vi "GetLeCroy_SaveToFile_25.vi"(1 "Digitizer Settings":T8={"Digitizer delay (us) "=0.0, "rf points per line"=2048, "lines per plane"=128, "Samp Rate (Hz)"=100000000.0, "Additional dig delay (us)"=0.0, "Voltage Scale"=0.4, "Pre-Looks"=0, "Offset delay (us)"=0.0, "bits A/D"=8, "Avg Num"=1, "DigTimeOut"=5.0, "Rel Dig Delay"=0.0, "Dig Ch"=0, "LeCroyCluster"={"LeCroy Channels"=[TRUE, FALSE, FALSE, FALSE], "LC read pt offset"=0.0, "Sweep Avg"=FALSE}, "Main Digitizer"=enum."NI Digitizer", "Dig Config"=enum."Single channel", "Digitizer ID Cluster"={"Acqiris/Alazar/SP ID"=[], "NI Instr Handles"=[], "LeCroy VISA"="", "GaGe Handle"={"Handle"=0, "Sample size"=0, "Resolution"=0, "Offset"=0, "Channels"=0, "Boards"=0}, "ATS Ref"="ATS9350", "Acqiris Address"=["PCI::INSTR0"], "ADQRef"=refnum, "adq_cu_ptr"=refnum}, "Trigger Settings"={"Trig Source"=1, "Trig Coupling"=0, "Trig Slope"=0, "Level (mV)"=1500.0}, "Bulk Acq"=FALSE, "Bulk Start Indexes"=[], "Data Ref RF"=refnum, "NI ID/Channel"=[], "Total Dig CH"=1, "Xtra Ann Trig delay (us)"=10.0, "Fix Z Delay?"=FALSE, "One Way Transmission?"=FALSE, "Data Ref Log"=refnum} {"Trigger Settings"."Trig Slope" items=["Positive", "Negative"]; "Trigger Settings"."Level (mV)" format="%.2f"; "Trigger Settings"."Trig Coupling" items=["DC 1 MOhm", "AC 1 MOhm", "DC 50 Ohm", "AC 50 Ohm"]; "Trigger Settings"."Trig Source" items=["Chan 1", "External"]; "Rel Dig Delay" format="%.2f"; "DigTimeOut" format="%.2f"; "Avg Num" min=1; "Offset delay (us)" format="%.2f"; "Additional dig delay (us)" format="%.2f"; "Digitizer delay (us)" format="%.2f"}, 4 "Ann Array Params":T1={"Synth Foc?"=FALSE, "Focal Zones"=41, "Switch T/R"=0, "Trans Geometry (mm)"={"Transducer"=0, "Geo Focus"=12.0, "a (radius)"=3.0, "# of rings"=5, "kerf space "=0.1, "Center Freq"=12.0}, "Sub Ap Excite?"=FALSE, "Full Array Scan?"=FALSE, "Xmt/Rcv"={"XMIT"=[TRUE, TRUE, TRUE, TRUE, TRUE], "RCV"=[TRUE, TRUE, TRUE, TRUE, TRUE]}, "PulseSpacing (us)"=0.0, "Xmit Ring"=0, "XMIT CHS"=0, "RCV CHS"=0, "GPU?"=FALSE, "Save TIFF?"=FALSE, "downfactor"=1, "RCV 1CH"=0} {"RCV 1CH" items=["All", "1", "2", "3", "4", "5"]; "Trans Geometry (mm)"."Transducer" items=["6D 12R 40 MHz"=0, "10D 31R 20 MHz"=1, "10D 23R 20 MHz"=2, "6D 23R 40 MHz"=3, "4.5D 10.7R 40 MHz"=4, "9D 23.5R 20 MHz"=5, "9D 25.8R 20MHz"=6, "Enter"=99]; "Switch T/R" min=1 max=5 step=1}, 5 "errorin":errorcluster, 6 "File Array":string[](array[string]), 7 "Motion Settings":T4={"No Motion?"=FALSE, "Motion System"=enum."NI 735x", "Motion Bd ID"=1, "Motion Profile"="SMAC1", "# Axis"=1, "Reverse Z axis?"=TRUE, "SMAC Axis"=0, "scan pair"=enum."y-(x) scan", "RT fps"=6.0, "Steps per mm"=[1000, 1000, 1000, 1000], "Motor Parameters"={"velocity ct/s"=[10000.0, 10000.0, 10000.0, 50000.0], "accel ct/s^2"=[50000.0, 50000.0, 50000.0, 200000.0]}, "One Way Scan"=FALSE, "Reverse One Way Scan"=FALSE, "Global Position (mm)"=[], "Plane"=0, "Distance between\nscan lines (um)"=0.0, "Distance between\nscan planes (um)"=0.0, "number of scan planes"=1, "Total steps in line"=0, "Xtra plane\ndistance  (um)"=100, "Xtra planes "=1, "Add Axis"=FALSE, "overshoot cts"=200, "BKPT Shift"=0, "Scan Start Time (ms)"=0, "ESP VISA"="GPIB::1::INSTR", "3rd Axis"=1, "GL Ref Out"=refnum, "Galil Address"=""} {"3rd Axis" items=["x", "y", "z", "w"]; "Xtra planes" min=1; "Xtra plane\ndistance  (um)" min=0; "Distance between\nscan planes (um)" format="%.2f"; "Distance between\nscan lines (um)" format="%.2f"; "SMAC Axis" items=["None"=0, "Axis 1"=1, "Axis 2"=2, "Axis 3"=3, "Axis 4"=4, "Axis 5"=5, "Axis 6"=6, "Axis 7"=7, "Axis 8"=8, "Vector Space 1"=17, "Vector Space 2"=18, "Vector Space 3"=19, "Vector Space 4"=20]; "Motion Bd ID" min=1 max=32 step=1}, 8 "lines per plane":i32, 11 "Reverse?":bool) -> (12 "Gain Array":T12(array[cluster]), 13 "Raw VGain (scale)":dbl, 15 "VGain (dB)":dbl, 19 "error out":errorcluster)   [LabVIEW 2022 SP3]
uses:
  -DigitizerRoutines/DigitizerSettings.ctl
  -DigitizerRoutines/Digitizer.ctl
  -DigitizerRoutines/DigConfig.ctl
  -DigitizerRoutines/DigitizerID.ctl
  C:/Windows/System32/ADQAPI_dotNet_helper.dll
  Motion Controllers/NI_controller/-NI_MotionRoutines/MotionParameters.ctl
  Motion Controllers/NI_controller/-NI_MotionRoutines/MotionSys.ctl
  Motion Controllers/-MotionRoutines/ScanAxis.ctl
  Motion Controllers/-MotionRoutines/3rdAxis.ctl
  Annular Array/-AnnularRoutines/AnnularArray.ctl
  Annular Array/-AnnularRoutines/TransGeometry.ctl
  Annular Array/-AnnularRoutines/ArrayGeometry.ctl
  Motion Controllers/-MotionRoutines/MotionGlobals.vi
  -ScanSystem/DataHandling/ReverseData.vi
panel:
  out "read time":u32
  out "save time":u32
  out "Numeric":i32
  # "1-D and 2-D B scan settings"
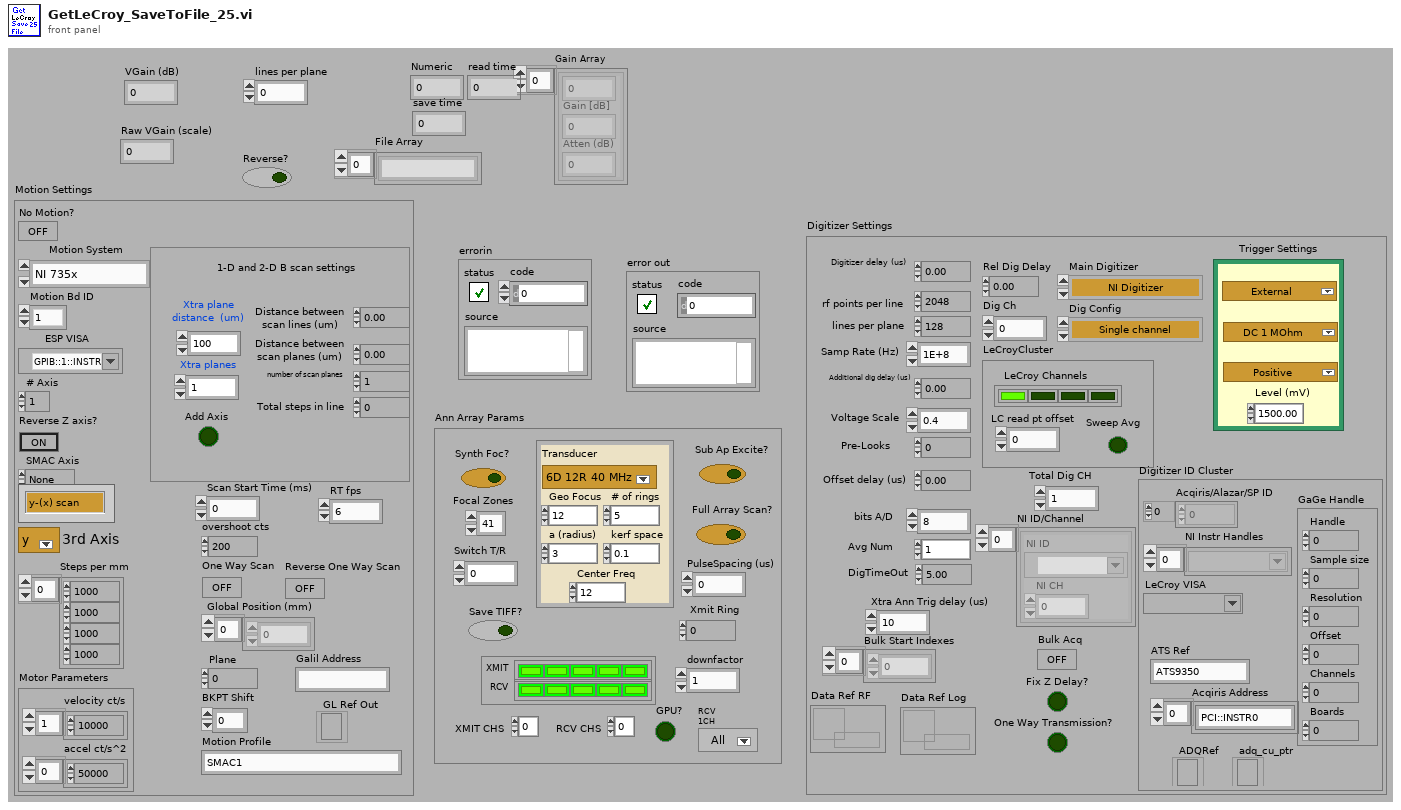
[diagram p1: front panel]
types:
  T1 = typedef "AnnularArray.ctl" = cluster{"Synth Foc?":bool, "Focal Zones":i16, "Switch T/R":i16, "Trans Geometry (mm)":T2, "Sub Ap Excite?":bool, "Full Array Scan?":bool, "Xmt/Rcv":cluster{"XMIT":bool[], "RCV":bool[]}, "PulseSpacing (us)":sgl, "Xmit Ring":i32, "XMIT CHS":u8, "RCV CHS":u8, "GPU?":bool, "Save TIFF?":bool, "downfactor":i32, "RCV 1CH":u16}
  T2 = typedef "TransGeometry.ctl" = cluster{"Transducer":T3, "Geo Focus":dbl, "a (radius)":dbl, "# of rings":i32, "kerf space ":dbl, "Center Freq":dbl}
  T3 = typedef "ArrayGeometry.ctl" = u16
  T4 = typedef "MotionParameters.ctl" = cluster{"No Motion?":bool, "Motion System":T5, "Motion Bd ID":u8, "Motion Profile":string, "# Axis":i8, "Reverse Z axis?":bool, "SMAC Axis":u16, "scan pair":T6, "RT fps":sgl, "Steps per mm":i32[], "Motor Parameters":cluster{"velocity ct/s":dbl[], "accel ct/s^2":dbl[]}, "One Way Scan":bool, "Reverse One Way Scan":bool, "Global Position (mm)":dbl[], "Plane":i32, "Distance between\nscan lines (um)":sgl, "Distance between\nscan planes (um)":sgl, "number of scan planes":i32, "Total steps in line":i32, "Xtra plane\ndistance  (um)":i32, "Xtra planes ":i32, "Add Axis":bool, "overshoot cts":i32, "BKPT Shift":i32, "Scan Start Time (ms)":u32, "ESP VISA":refnum<visa-resource-name>, "3rd Axis":T7, "GL Ref Out":refnum<k7>, "Galil Address":string}
  T5 = typedef "MotionSys.ctl" = enum16{"MM3000", "NI 735x", "Newport ESP", "No Motion Card", "Galil"}
  T6 = typedef "ScanAxis.ctl" = enum16{"y-(x) scan", "x-(y) scan", "z-(x) scan", "z-(y) scan", "y-(z) scan", "x-(z) scan", "w-(x) scan", "w-(y) scan", "w-(z) scan", "x-(w) scan", "y-(w) scan", "z-(w) scan"}
  T7 = typedef "3rdAxis.ctl" = u16
  T8 = typedef "DigitizerSettings.ctl" = cluster{"Digitizer delay (us) ":dbl, "rf points per line":i32, "lines per plane":i32, "Samp Rate (Hz)":dbl, "Additional dig delay (us)":dbl, "Voltage Scale":dbl, "Pre-Looks":i32, "Offset delay (us)":dbl, "bits A/D":i8, "Avg Num":i32, "DigTimeOut":sgl, "Rel Dig Delay":sgl, "Dig Ch":i32, "LeCroyCluster":cluster{"LeCroy Channels":bool[], "LC read pt offset":dbl, "Sweep Avg":bool}, "Main Digitizer":T9, "Dig Config":T10, "Digitizer ID Cluster":T11, "Trigger Settings":cluster{"Trig Source":u16, "Trig Coupling":u16, "Trig Slope":u16, "Level (mV)":dbl}, "Bulk Acq":bool, "Bulk Start Indexes":i32[], "Data Ref RF":refnum<data-value>, "NI ID/Channel":cluster{"NI ID":refnum<k15>, "NI CH":i32}[], "Total Dig CH":i32, "Xtra Ann Trig delay (us)":dbl, "Fix Z Delay?":bool, "One Way Transmission?":bool, "Data Ref Log":refnum<data-value>}
  T9 = typedef "Digitizer.ctl" = enum16{"Acqiris Digitizer", "NI Digitizer", "LeCroy", "GaGe", "AlazarTech", "No Digitizer", "Teledyne"}
  T10 = typedef "DigConfig.ctl" = enum16{"Single channel", "2 Chans w/ 2 Acqiris", "2 Chans w/ 1 Acqiris", "5-CH Pulser New", "5-CH pulser w/ ann array", "5-pass style ann array", "Empty"}
  T11 = typedef "DigitizerID.ctl" = cluster{"Acqiris/Alazar/SP ID":u32[], "NI Instr Handles":refnum<k15>[], "LeCroy VISA":refnum<visa-resource-name>, "GaGe Handle":cluster{"Handle":u32, "Sample size":u32, "Resolution":i32, "Offset":i32, "Channels":u32, "Boards":u32}, "ATS Ref":string, "Acqiris Address":string[], "ADQRef":refnum<k24>, "adq_cu_ptr":refnum<k24>}
  T12 = cluster{sgl, "Gain [dB]  ":sgl, "Atten (dB)":sgl}[]
  T13 = cluster{"wfm":i16[][], "max queue size (-1, unlimited)":i32, "Voltage Scale":cluster{sgl, "Gain [dB]  ":sgl, "Atten (dB)":sgl}}
  T14 = enum16{"open", "replace", "create", "open or create", "replace or create", "replace or create with confirmation"}
  T15 = enum16{"big-endian, network order", "native, host order", "little-endian"}
  T16 = cluster{sgl, "Gain [dB]  ":sgl, "Atten (dB)":sgl}
  T17 = cluster{i16[][], i32, "Voltage Scale":cluster{sgl, "Gain [dB]  ":sgl, "Atten (dB)":sgl}}
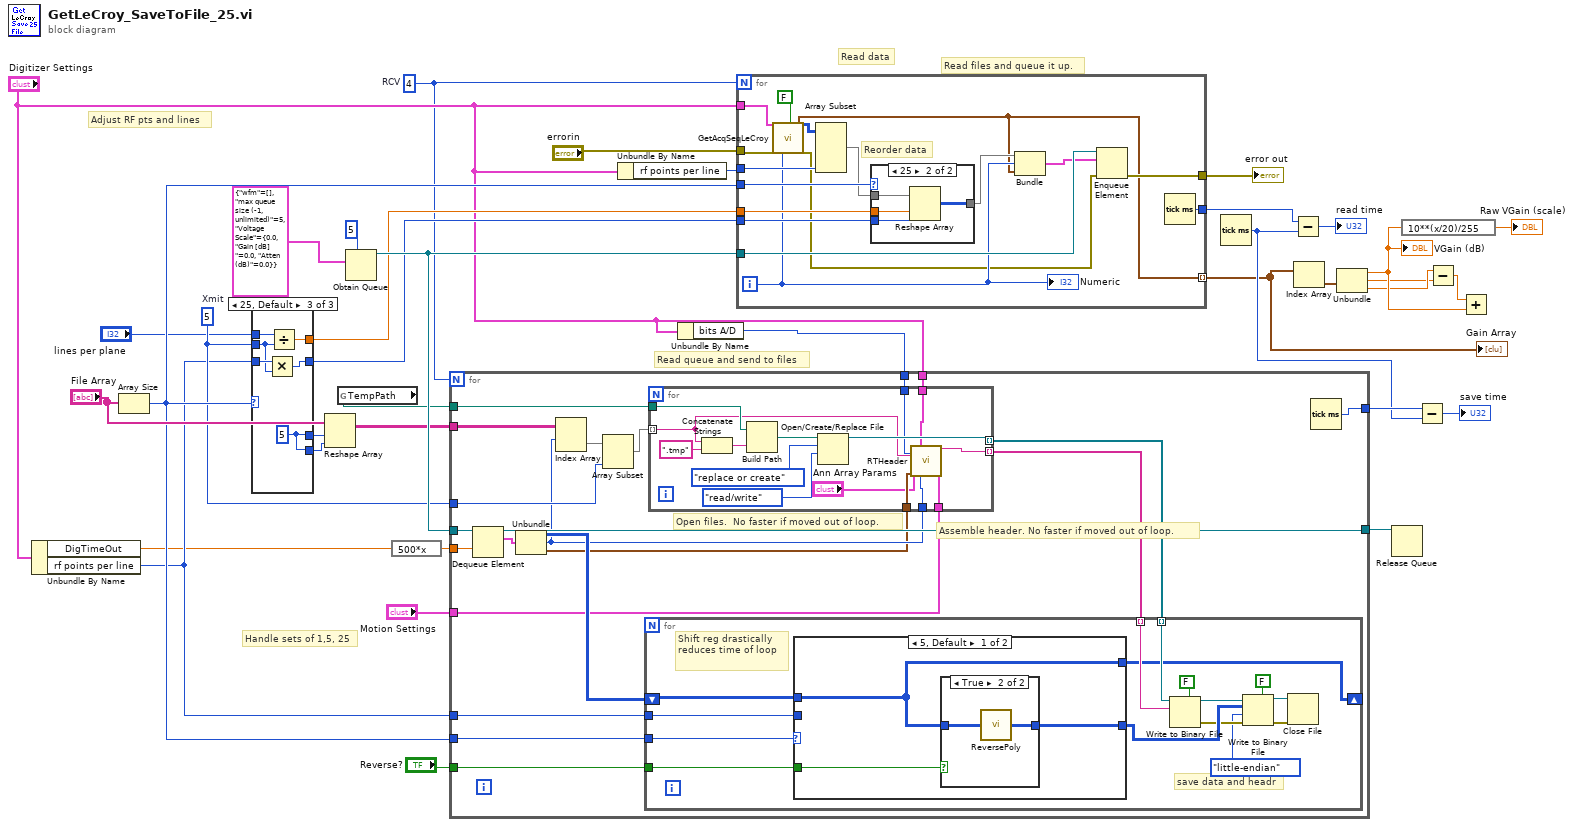
[diagram p0: block diagram]
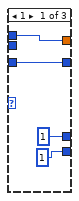
[diagram p3: hidden frame]
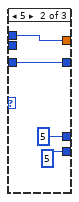
[diagram p4: hidden frame]
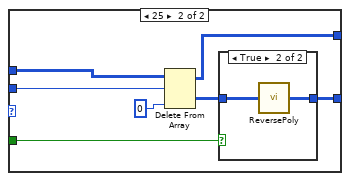
[diagram p6: hidden frame]
diagram:
  w12 = 5  # Xmit
  w3 = 4  # RCV
  # "Read files and queue it up."
  # "Read data"
  # "Adjust RF pts and lines"
  # "Handle sets of 1,5, 25"
  # "Read queue and send to files"
  n1 = Unbundle By Name("Digitizer Settings") -> ("DigTimeOut"=w10:sgl, "rf points per line"=w11:i32)
  n2 = Array Size(array="File Array") -> (size(s)=w15:i32)
  n3 = case shown="25, Default" w15 {
    tunnel: [1 5 w51] -> w20
    tunnel: [w40 w44 w47] -> w17
    tunnel: w11 -> [w40 w44 w48]
    tunnel: [w39 w43 w49] -> w18
    tunnel: "lines per plane" -> [w39 w43 w50]
    tunnel: [1 5 w51] -> w19
    tunnel: w12 -> [_ _ w46]
    frame 1 {
    }
    frame 5 {
    }
    frame 25, Default {
      w51 = 5
      n4 = Multiply(x=w48, y=w46) -> (x*y=w47:i32)
      n5 = Divide(x=w50, y=w46) -> (x/y=w49:dbl)
    }
  }
  n6 = Reshape Array("File Array", w20, w19) -> (w14:string[][])
  n7 = global read "MotionGlobals.vi" "TempPath"() -> (w13:path)
  n8 = Obtain Queue(max queue size (-1, unlimited)=5, element data type=T13 {"wfm"=[], "max queue size (-1, unlimited)"=5, "Voltage Scale"={0.0, "Gain [dB]  "=0.0, "Atten (dB)"=0.0}}) -> (queue out=w30:refnum<queue>)  [unwired: 3 in, 2 out]
  n9 = expression code="500*x"(w10) -> (w16:sgl)
  n10 = Unbundle By Name("Digitizer Settings") -> ("rf points per line"=w7:i32)
  n11 = Unbundle By Name("Digitizer Settings") -> ("bits A/D"=w1:i8)
  n12 = for {
    N: w3 -> [_]
    tunnel: w11 -> [w72]
    tunnel: "Reverse?" -> [w67]
    tunnel: w30 -> [w71]
    tunnel: [w69] -> w22
    tunnel: [w68] -> w27
    tunnel: w15 -> [w66]
    tunnel: w16 -> [w65]
    tunnel: w14 -> [w60]
    tunnel: w13 -> [w63]
    tunnel: w1 -> [w62]
    tunnel: w12 -> [w57]
    tunnel: "Digitizer Settings" -> [w55]
    tunnel: "Motion Settings" -> [w54]
    # "Open files.  No faster if moved out of loop."
    # "Assemble header. No faster if moved out of loop."
    n13 = Dequeue Element(queue=w71, timeout in ms (-1)=w65) -> (queue out=w69:refnum<queue>, element=w70:T13)  [unwired: 1 in, 2 out]
    n14 = Unbundle(w70) -> ("wfm"=w56:i16[][], "max queue size (-1, unlimited)"=w53:i32, "Voltage Scale"=w52:T16)
    n15 = Index Array(array=w60, index (row)=w53) -> (element=w58:string[])  [unwired: 1 in]
    n16 = Array Subset(array=w58, length=w57) -> (w59:string[])  [unwired: 1 in]
    n17 = for {
      tunnel: w59 -> [w80] mode=indexing
      tunnel: [w82] -> w64 mode=indexing
      tunnel: w63 -> [w81]
      tunnel: w52 -> [w79]
      tunnel: w62 -> [w78]
      tunnel: [w77] -> w61 mode=indexing
      tunnel: w55 -> [w76]
      tunnel: w54 -> [w75]
      tunnel: w53 -> [w74]
      n18 = Concatenate Strings(w80, ".tmp") -> (w83:string)
      n19 = Build Path(base path=w81, name or relative path=w83) -> (appended path=w87:path)
      n20 = Open/Create/Replace File(file path (use dialog)=w87, operation (0:open)=T14."replace or create", access (0:read/write)=enum16{"read/write", "read-only", "write-only"}."read/write") -> (refnum out=w82:refnum<file>)  [unwired: 1 in, 4 out]
      n21 = call "RTHeader.vi"("Digitizer Settings"=w76, "Dig Word Size"=w78, "File Name In"=w80, "Ann Array Params"="Ann Array Params", "Votage scaling"=w79, "Pulser Channel"=w74, "Motion Settings"=w75) -> ("Header String Out"=w77:string)  [unwired: 7 in, 1 out]
    }
    n22 = for {
      tunnel: w61 -> [w100] mode=indexing
      tunnel: w67 -> [w99]
      tunnel: w64 -> [w92] mode=indexing
      tunnel: w72 -> [w98]
      tunnel: w66 -> [w96]
      shift-right: [w89] -> _
      shift-left: w56 -> [w97]
      # "Shift reg drastically reduces time of loop"
      # "save data and headr"
      n23 = case shown="5, Default" w96 {
        tunnel: w99 -> [w105 w113]
        tunnel: [w104 w114] -> w95
        tunnel: w98 -> [_ w110]
        tunnel: w97 -> [w103 w112]
        tunnel: [w103 w111] -> w89
        frame 5, Default {
          n24 = case shown="True" w105 {
            tunnel: [w106 w108] -> w104
            tunnel: w103 -> [w106 w107]
            frame False {
            }
            frame True {
              n25 = call-poly "ReversePoly.vi"("Array in"=w107) -> ("Array out"=w108:i16[][])
            }
          }
        }
        frame 25 {
          n26 = Delete From Array(array=w112, length=w110, index (col)=0 ("index (row)")) -> (deleted portion=w115:i16[][], array with subset deleted=w111:i16[][])  [unwired: 1 in]
          n27 = case shown="True" w113 {
            tunnel: [w116 w118] -> w114
            tunnel: w115 -> [w116 w117]
            frame False {
            }
            frame True {
              n28 = call-poly "ReversePoly.vi"("Array in"=w117) -> ("Array out"=w118:i16[][])
            }
          }
        }
      }
      n29 = Write to Binary File(file (use dialog)=w92, data=w100, 5:FALSE ("prepend array or string size? (T)")) -> (refnum out=w91:refnum<file>, error out=w90:errorcluster)  [unwired: 3 in, 1 out]
      n30 = Write to Binary File(file (use dialog)=w91, data=w95, error in=w90, 5:FALSE ("prepend array or string size? (T)"), 9:T15."little-endian" ("byte order (0:big-endian, network order)")) -> (refnum out=w94:refnum<file>, error out=w93:errorcluster)  [unwired: 1 in, 1 out]
      n31 = Close File(refnum=w94, error in=w93) -> ()  [unwired: 2 out]
    }
    n32 = Tick Count (ms)() -> (millisecond timer value=w68:u32)
  }
  n33 = for {
    N: w3 -> [_]
    tunnel: w30 -> [w135]
    tunnel: [w133] -> w28
    tunnel: [w132] -> w6
    tunnel: w15 -> [w131]
    tunnel: w18 -> [w130]
    tunnel: w17 -> [w129]
    tunnel: w7 -> [w127]
    tunnel: "errorin" -> [w124]
    tunnel: "Digitizer Settings" -> [w123]
    tunnel: [w120] -> w2 mode=indexing
    i -> [w121]
    # "Reorder data"
    n34 = call "GetAcqSeqLeCroy.vi"("Digitizer Settings"=w123, "errorin"=w124, "Source (0: Channel 1)"=w121, "save?"=FALSE) -> ("Voltage Scale"=w120:T16, "Data Array"=w125:i16[][], "error out"=w119:errorcluster)  [unwired: 17 in, 4 out]
    n35 = Array Subset(array=w125, length (col)=w127) -> (w126:i16[][])  [unwired: 3 in]
    n36 = case shown="25" w131 {
      tunnel: w129 -> [_ w140]
      tunnel: w126 -> [w136 w139]
      tunnel: [w136 w138] -> w128
      tunnel: w130 -> [_ w137]
      frame 0, Default {
      }
      frame 25 {
        n37 = Reshape Array(w139, w137, w140) -> (w138:i16[][])
      }
    }
    n38 = Bundle(w128, w121, "Voltage Scale"=w120) -> (w134:T17)  [unwired: 1 in]
    n39 = Enqueue Element(queue=w135, element=w134, error in (no error)=w119) -> (error out=w132:errorcluster)  [unwired: 1 in, 2 out]
    n40 = Tick Count (ms)() -> (millisecond timer value=w133:u32)
    "Numeric" <- w121
  }
  "error out" <- w6
  "Gain Array" <- w2
  n41 = Tick Count (ms)() -> (millisecond timer value=w26:u32)
  n42 = Subtract(x=w28, y=w26) -> (x-y=→"read time":u32)
  n43 = Index Array(array=w2) -> (element=w37:T16)  [unwired: 1 in]
  n44 = Unbundle(w37) -> (w36:sgl, "Gain [dB]"=w34:sgl, "Atten (dB)"=w35:sgl)
  "VGain (dB)" <- w36
  n45 = Release Queue(queue=w22) -> ()  [unwired: 2 in, 3 out]
  n46 = expression code="10**(x/20)/255"(w36) -> (→"Raw VGain (scale)":sgl)
  n47 = Subtract(x=w27, y=w26) -> (x-y=→"save time":u32)
  n48 = Subtract(x=w35, y=w34) -> (x-y=w33:sgl)
  n49 = Add(x=w33, y=w36) -> ()  [unwired: 1 out]
